vi "TDMS image save.vi"(7 "Save Image Path":path, 8 "error in (no error)":errorcluster, 9 "Status":T3, 11 "Refnum in":T2) -> (0 "error out":errorcluster)   [LabVIEW 2020, in "Point Grey Camera.lvclass"]
uses:
  Point Grey Camera.lvclass
  1st or last shot of scan.ctl
  <vilib>/vision/Image Controls.llb/IMAQ Image.ctl
  <userlib>/_OpenG.lib/file/file.llb/Strip Path Extension - Path__ogtk.vi
  <resource>/objmgr/IMAQImage.rc
panel:
  out "Image Type 2":T1 items=["Grayscale (U8)", "Grayscale (I16)", "Grayscale (SGL)", "Complex (CSG)", "RGB (U32)", "HSL (U32)", "RGB (U64)", "Grayscale (U16)"]
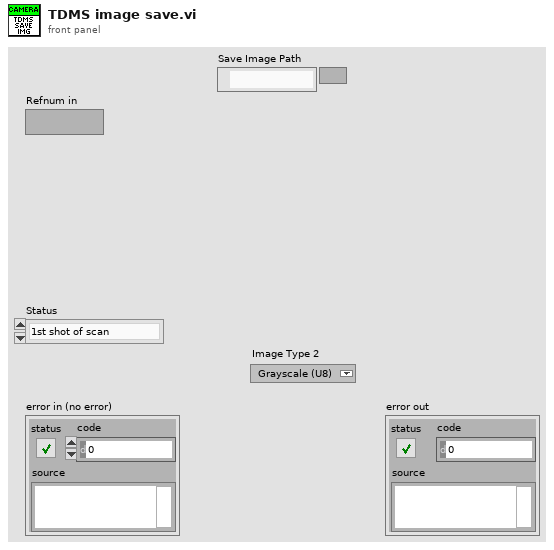
[diagram p1: front panel]
types:
  T1 = typedef "Image Type" = u32
  T2 = typedef "IMAQ Image.ctl" = refnum<image>
  T3 = typedef "1st or last shot of scan.ctl" = enum16{"1st shot of scan", "1st shot after scan end", "other"}
  T4 = enum16{"open", "open or create", "create or replace", "create", "open (read-only)"}
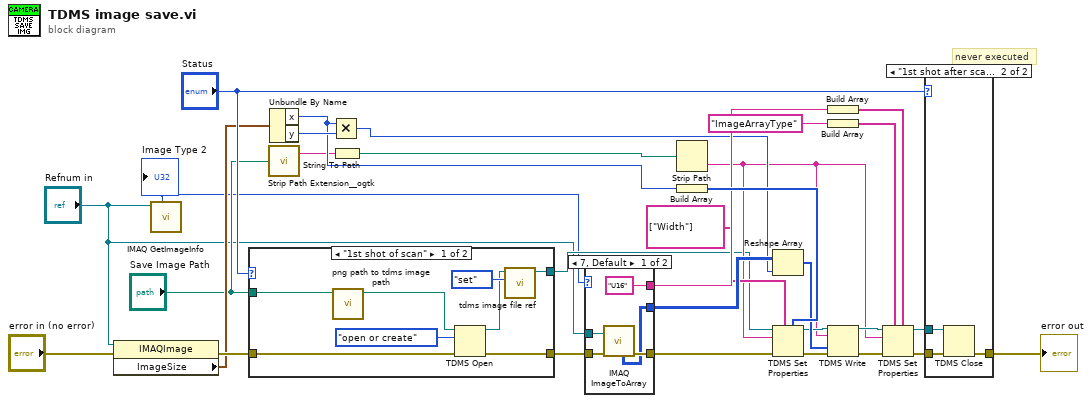
[diagram p0: block diagram]
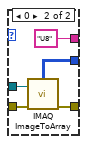
[diagram p3: hidden frame]
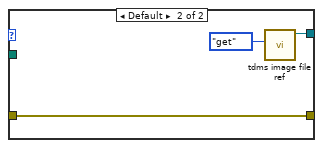
[diagram p4: hidden frame]
diagram:
  # "never executed"
  n1 = property class="IMAQImage"(reference="Refnum in", error in="error in (no error)") -> (error out=w30:errorcluster, "ImageSize"=w25:cluster{"x":i32, "y":i32})  [unwired: 1 out]
  n2 = call "IMAQ GetImageInfo"("Image"="Refnum in") -> ("Image Type"=w1:T1)  [unwired: 3 in, 7 out]
  "Image Type 2" <- w1
  n3 = case shown="\"1st shot of scan\"" "Status" {
    tunnel: [w34 w41] -> w3
    tunnel: w30 -> [w38 w42]
    tunnel: [w37 w42] -> w4
    tunnel: "Save Image Path" -> [w33 _]
    frame "1st shot of scan" {
      n4 = call "png path to tdms image path.vi"("png path"=w33) -> ("tdms image path"=w32:path)  [unwired: 7 in, 3 out]
      n5 = TDMS Open(8:w38, 10:T4."open or create" ("operation (0:open)"), 11:w32) -> (0:w37:errorcluster, 3:w35:refnum<k34>)  [unwired: 4 in]
      n6 = call "tdms image file ref.vi"("command"=enum16{"set", "get"}."set", "tdms file ref"=w35) -> ("tdms file ref"=w34:refnum<k34>)  [unwired: 9 in]
    }
    frame Default {
      n7 = call "tdms image file ref.vi"("command"=enum16{"set", "get"}."get") -> ("tdms file ref"=w41:refnum<k34>)  [unwired: 10 in]
    }
  }
  n8 = call-poly <userlib>:"Strip Path Extension__ogtk.vi"("path"="Save Image Path") -> ("root"=w10:string)  [unwired: 1 out]
  n9 = Unbundle By Name(w25) -> ("x"=w28:i32, "y"=w29:i32)
  n10 = Multiply(x=w28, y=w29) -> (x*y=w17:i32)
  n11 = String To Path(string=w10) -> (path=w11:path)
  n12 = case shown="7, Default" w1 {
    tunnel: "Refnum in" -> [w47 w52]
    tunnel: w4 -> [w46 w51]
    tunnel: [w45 w50] -> w19
    tunnel: [w44 w49] -> w23
    tunnel: ["U16" "U8"] -> w24
    frame 7, Default {
      n13 = call "IMAQ ImageToArray"("error in (no error)"=w46, "Image"=w47) -> ("Image Pixels (U16)"=w44:u16[][], "error out"=w45:errorcluster)  [unwired: 2 in, 3 out]
    }
    frame 0 {
      n14 = call "IMAQ ImageToArray"("error in (no error)"=w51, "Image"=w52) -> ("error out"=w50:errorcluster, "Image Pixels (U8)"=w49:u8[][])  [unwired: 2 in, 3 out]
    }
  }
  n15 = Strip Path(path=w11) -> (name=w9:string)  [unwired: 1 out]
  n16 = Build Array(w28) -> (w27:i32[])
  n17 = Reshape Array(w23, w17) -> (w18:u16[])
  n18 = TDMS Set Properties(5:w27, 7:string[] ["Width"] ("property names"), 8:w19, 10:w9, 11:w3) -> (0:w14:errorcluster, 3:w13:refnum<k34>)  [unwired: 1 in, 2 out]
  n19 = Build Array(w24) -> (w20:string[])
  n20 = Build Array("ImageArrayType") -> (w22:string[])
  n21 = TDMS Write(0:w13, 5:w9, 9:w18, 11:w14) -> (4:w15:refnum<k34>, 15:w16:errorcluster)  [unwired: 2 in, 2 out]
  n22 = TDMS Set Properties(5:w20, 7:w22, 8:w16, 10:w9, 11:w15) -> (0:w6:errorcluster, 3:w5:refnum<k34>)  [unwired: 1 in, 2 out]
  n23 = case shown="\"1st shot after scan end\"" "Status" {
    tunnel: w5 -> [_ w56]
    tunnel: w6 -> [w53 w55]
    tunnel: [w53 w54] -> w8
    frame "1st shot of scan", Default {
    }
    frame "1st shot after scan end" {
      n24 = TDMS Close(8:w55, 11:w56) -> (0:w54:errorcluster)  [unwired: 1 out]
    }
  }
  "error out" <- w8
